vi "Fibonaci Calculator demo.vi"() -> ()   [LabVIEW 2013]
panel:
  out "i":i32
  out "element":enum16{"Stop", "Proceed"}(ring)
  in  "Stop Button":bool
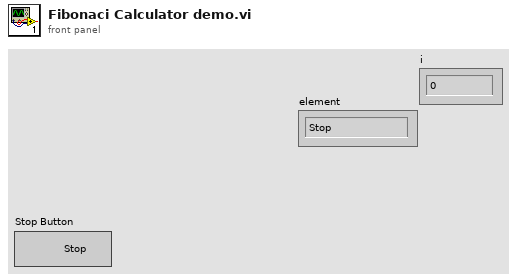
[diagram p1: front panel]
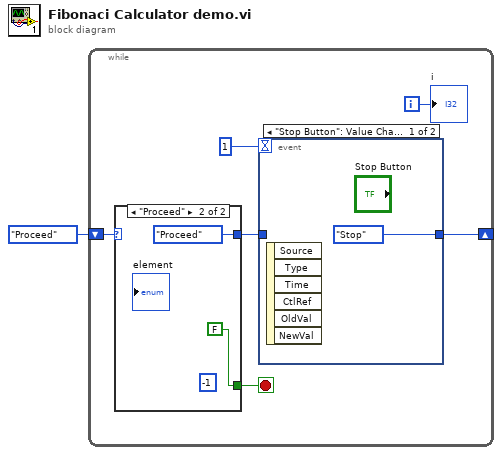
[diagram p0: block diagram]
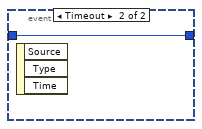
[diagram p2: hidden frame]
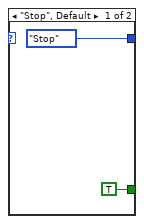
[diagram p3: hidden frame]
diagram:
  n1 = while {
    shift-right: [w3] -> _
    shift-left: enum16{"Stop", "Proceed"}."Proceed" -> [w7]
    i -> [w5]
    stop <- w6 stop-if-true
    n2 = case shown="\"Proceed\"" w7 {
      tunnel: [enum16{"Stop", "Proceed"}."Stop" enum16{"Stop", "Proceed"}."Proceed"] -> w4
      tunnel: [TRUE FALSE] -> w6
      frame "Stop", Default {
      }
      frame "Proceed" {
        (unwired) -1 ("timeout in ms (-1)")
      }
    }
    n3 = event shown="[0] \"Stop Button\": Value Change" {
      selector: _ -> [_ _]
      dyn-events: _ -> [_ _]
      timeout: 1 -> [_ _]
      tunnel: [enum16{"Stop", "Proceed"}."Stop" w9] -> w3
      tunnel: w4 -> [_ w9]
      event "Stop Button": Value Change {
        n4 = event-data() -> ()  [unwired: 1 in, 6 out]
      }
      event Timeout {
        n5 = event-data() -> ()  [unwired: 1 in, 3 out]
      }
    }
    "i" <- w5
  }
